vi "PublishCurrentValues.vi"(7 "DataGroups ChannelStatus":T1[](array[typedef]), 8 "error in (no error)":errorcluster, 10 "Qbus in":refnum<class "Qbus.lvclass">, 11 "config in":T3) -> (0 "error out":errorcluster, 3 "config out":T3)   [LabVIEW 2017, in "McsaTestPanel.lvlib"]
uses:
  <vilib>/addons/InsightCM/Devices/Shared/Mcsa/McsaTestPanel/McsaTestPanel.lvlib
  <vilib>/addons/InsightCM/Devices/Shared/Common/TestPanel/controls/Configuration.ctl
  <vilib>/addons/InsightCM/Devices/Shared/Common/TestPanel/controls/State.ctl
  <vilib>/addons/InsightCM/MessageBus/Base/controls/IRoutingSource.ctl
  <vilib>/addons/Qbus/Qbus.lvclass
  <vilib>/addons/InsightCM/Devices/Shared/Mcsa/McsaTestPanel/controls/ChannelStatus.ctl
  <vilib>/addons/InsightCM/MessageBus/Base/controls/KeyValuePair.ctl
  <vilib>/addons/InsightCM/MessageBus/MessageLibrary/Device/controls/DeviceTestPanelGetCurrentValuesResponseBody.ctl
  <vilib>/addons/InsightCM/MessageBus/Base/controls/TestPanelCurrentValues.ctl
  <vilib>/addons/InsightCM/MessageBus/Base/controls/TestPanelCurrentValue.ctl
  <vilib>/addons/InsightCM/MessageBus/Base/controls/TestPanelValue.ctl
  <vilib>/addons/InsightCM/Devices/Shared/Common/TestPanel/TestPanel.lvlib
  <vilib>/addons/InsightCM/Devices/Shared/Common/ServerComm/ServerComm.lvlib
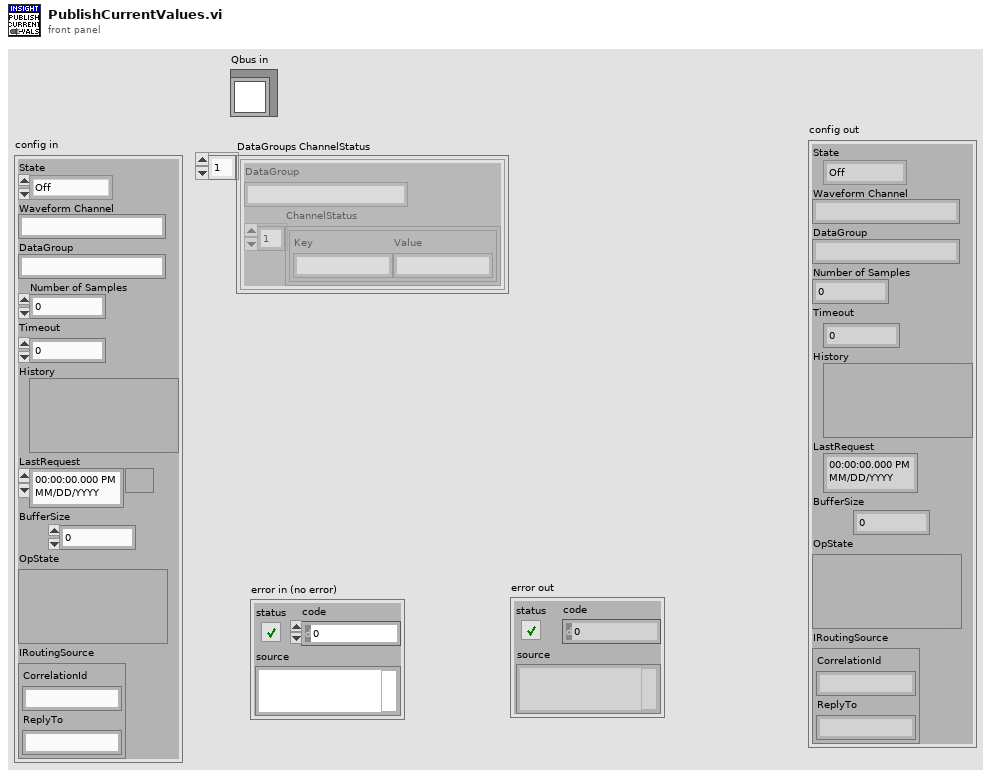
[diagram p1: front panel]
types:
  T1 = typedef "McsaTestPanel.lvlib/ChannelStatus.ctl" = cluster{"DataGroup":string, "ChannelStatus":T2[]}
  T2 = typedef "KeyValuePair.ctl" = cluster{"Key":string, "Value":string}
  T3 = typedef "TestPanel.lvlib/Configuration.ctl" = cluster{"State":T4, "Waveform Channel":string, "DataGroup":string, "Number of Samples":i32, "Timeout":dbl, "History":variant, "LastRequest":timestamp, "BufferSize":i32, "OpState":variant, "IRoutingSource":T5}
  T4 = typedef "TestPanel.lvlib/State.ctl" = enum16{"Off", "On", "PendingValues", "PendingDataSet"}
  T5 = typedef "IRoutingSource.ctl" = cluster{"CorrelationId":string, "ReplyTo":string}
  T6 = typedef "DeviceTestPanelGetCurrentValuesResponseBody.ctl" = cluster{"Data":T7[]}
  T7 = typedef "TestPanelCurrentValues.ctl" = cluster{"DataGroup":string, "OperatingState":string, "ChannelStatus":T2[], "Values":T8[]}
  T8 = typedef "TestPanelCurrentValue.ctl" = cluster{"TrendPointId":string, "AssetName":string, "MetricName":string, "Unit":string, "Value":T9}
  T9 = typedef "TestPanelValue.ctl" = cluster{"Value":dbl, "Timestamp":i64, "Invalid":bool}
  T10 = typedef "Message.ctl" = cluster{"Header":T11, "Body":u8[]}
  T11 = typedef "MessageHeader.ctl" = cluster{"MessageName":string, "Timestamp":i64, "CorrelationId":string, "ContentType":string, "RoutingKey":string, "Properties":T2[]}
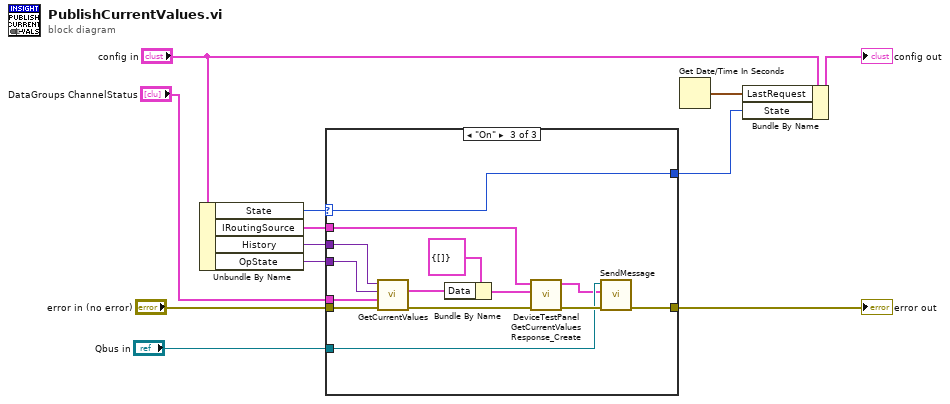
[diagram p0: block diagram]
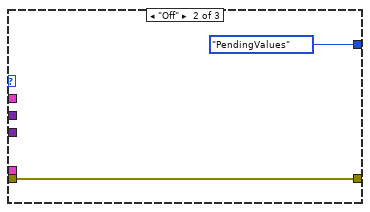
[diagram p3: hidden frame]
diagram:
  n1 = Unbundle By Name("config in") -> ("State"=w9:T4, "IRoutingSource"=w5:T5, "History"=w8:variant, "OpState"=w7:variant)
  n2 = case shown="\"On\"" w9 {
    selector: w9 -> [w14 _ w22]
    tunnel: w8 -> [_ _ w30]
    tunnel: w7 -> [_ _ w29]
    tunnel: "error in (no error)" -> [w13 w15 w25]
    tunnel: w5 -> [_ _ w23]
    tunnel: "Qbus in" -> [_ _ w18]
    tunnel: [w13 w15 w19] -> w3
    tunnel: [w14 State."PendingValues" ("State") w22] -> w2
    tunnel: "DataGroups ChannelStatus" -> [_ _ w21]
    frame Default {
    }
    frame "Off" {
    }
    frame "On" {
      n3 = call <vilib>:"GetCurrentValues.vi"("error in (no error)"=w25, "DataGroups ChannelStatus"=w21, "OpState"=w29, "History"=w30) -> ("error out"=w24:errorcluster, "current values"=w27:T7[])  [unwired: 6 in]
      n4 = Bundle By Name(cluster=T6 {"Data"=[]} ("DeviceTestPanelGetCurrentValuesResponse"), "Data"=w27) -> (w26:T6)
      n5 = call <vilib>:"DeviceTestPanelGetCurrentValuesResponse_Create.vi"("error in (no error)"=w24, "DeviceTestPanelGetCurrentValuesResponse"=w26, "IRoutingSource"=w23) -> ("error out"=w20:errorcluster, "Message"=w17:T10)  [unwired: 7 in]
      n6 = call <vilib>:"SendMessage.vi"("error in (no error)"=w20, "message"=w17, "Qbus in"=w18) -> ("error out"=w19:errorcluster)  [unwired: 7 in, 1 out]
    }
  }
  "error out" <- w3
  n7 = Get Date/Time In Seconds() -> (seconds since 1Jan1904=w10:timestamp)
  n8 = Bundle By Name(cluster="config in", "LastRequest"=w10, "State"=w2) -> (→"config out":T3)
